vi "pulse_from_trigger.vi"(10 "trigger":bool, 11 "Pulse width":u16) -> (2 "count":u16, 3 "pulse":bool)   [LabVIEW 2017]
uses:
  <instrlib>/_niInstr/Basic Elements/v1/FPGA/niInstr Basic Elements v1 FPGA.lvlib
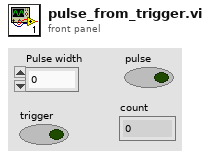
[diagram p1: front panel]
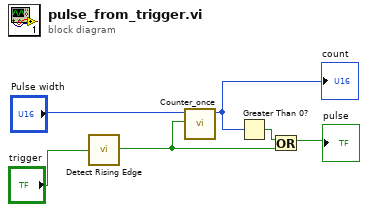
[diagram p0: block diagram]
diagram:
  n1 = call <instrlib>:"Detect Rising Edge.vi"("signal"="trigger") -> ("edge detected"=w4:bool)  [unwired: 14 in]
  n2 = call "Counter_once.vi"("reset"=w4, "limit"="Pulse width") -> ("count"=w3:u16)  [unwired: 9 in]
  "count" <- w3
  n3 = Greater Than 0?(x=w3) -> (x > 0?=w2:bool)
  n4 = Or(x=w2, y=w4) -> (x .or. y?=→"pulse":bool)
